vi "Combine Values.vi"(8 "error in":errorcluster, 10 "New Values":dbl[][](array[numeric]), 11 "Old Values":dbl[][][](array[numeric])) -> (0 "error out":errorcluster, 3 "Combined Values":dbl[][][](array[numeric]))   [LabVIEW 2017, in "Akwizycja.lvlib"]
uses:
  Akwizycja.lvlib
  <vilib>/Utility/config.llb/NI_LVConfig.lvlib
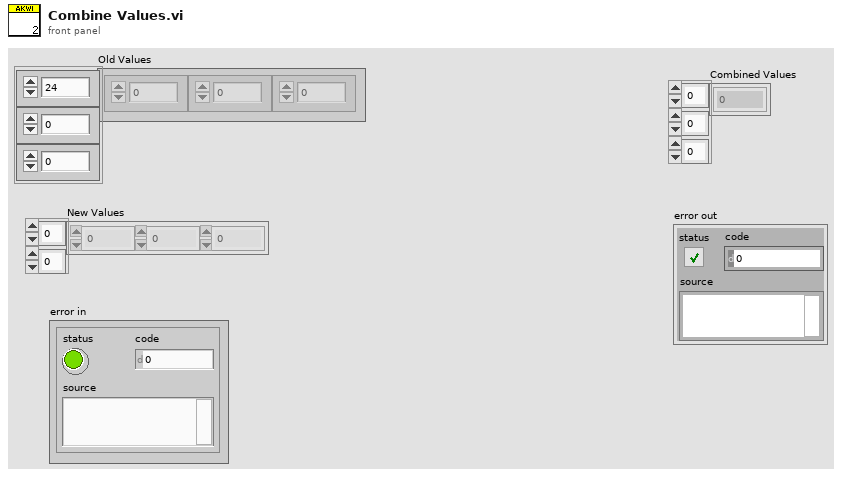
[diagram p1: front panel]
types:
  T1 = typedef "NI_LVConfig.lvlib/Config Data RefNum.ctl" = refnum<k1>
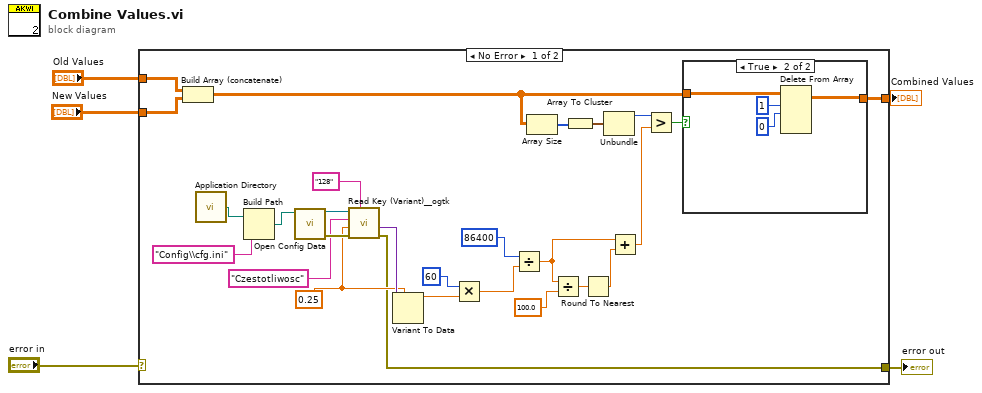
[diagram p0: block diagram]
diagram:
  n1 = case shown="No Error" "error in" {
    selector: "error in" -> [_ w38]
    tunnel: "New Values" -> [w27 _]
    tunnel: "Old Values" -> [w28 w39]
    tunnel: [w25 w39] -> w2
    tunnel: [w6 w38] -> w1
    frame No Error {
      w15 = 0.25
      n2 = Build Array (concatenate)(w28, w27) -> (w26:dbl[][][])
      n3 = call <vilib>:"Application Directory.vi"() -> ("Application Directory"=w22:path)
      n4 = Build Path(base path=w22, name or relative path="Config\\cfg.ini") -> (appended path=w21:path)
      n5 = call <vilib>:"Open Config Data.vi"("configuration file path"=w21) -> ("error out"=w19:errorcluster, "refnum"=w20:T1)  [unwired: 8 in, 1 out]
      n6 = call <userlib>:"Read Key (Variant)__ogtk.vi"("section"="128", "error in (no error)"=w19, "type"=w15, "key (optional)"="Czestotliwosc", "refnum"=w20) -> ("error out"=w6:errorcluster, "key-value"=w18:variant)  [unwired: 3 in, 2 out]
      n7 = Variant To Data(type=w15, Variant=w18) -> (data=w23:dbl)  [unwired: 1 in, 1 out]
      n8 = Multiply(x=60, y=w23) -> (x*y=w24:dbl)
      n9 = Divide(x=86400, y=w24) -> (x/y=w11:dbl)
      n10 = Array Size(array=w26) -> (size(s)=w29:i32[])
      n11 = Divide(x=w11, y=100.0) -> (x/y=w9:dbl)
      n12 = Array To Cluster(array=w29) -> (cluster=w30:cluster{"[0]":i32, "[1]":i32, "[2]":i32})
      n13 = Round To Nearest(number=w9) -> (nearest integer value=w8:dbl)
      n14 = Unbundle(w30) -> ("[0]"=w31:i32)  [unwired: 2 out]
      n15 = Add(x=w11, y=w8) -> (x+y=w7:dbl)
      n16 = Greater?(x=w31, y=w7) -> (0:w32:bool)
      n17 = case shown="True" w32 {
        tunnel: w26 -> [w33 w36]
        tunnel: [w33 w35] -> w25
        frame False {
        }
        frame True {
          n18 = Delete From Array(array=w36, length=1, index (dim 0)=0 ("index (page)")) -> (array with subset deleted=w35:dbl[][][])  [unwired: 2 in, 1 out]
        }
      }
    }
    frame Error {
    }
  }
  "Combined Values" <- w2
  "error out" <- w1
